vi "SLL Get Graph and File Sampling Rate.vi"(8 "error in (no error)":errorcluster) -> (0 "error out":errorcluster, 1 "File - Interval b/w Samples":i32, 2 "Graph - Interval b/w Samples":i32, 3 "AI Sampling Rate (Samples/Sec)":dbl)   [LabVIEW 2013]
doc: "Copyright © 2005, Soliton Technologies.\nAll rights reserved."
uses:
  DAQ Engine/Controls/SLL DE DAQ Parameters LV2Global Options.ctl
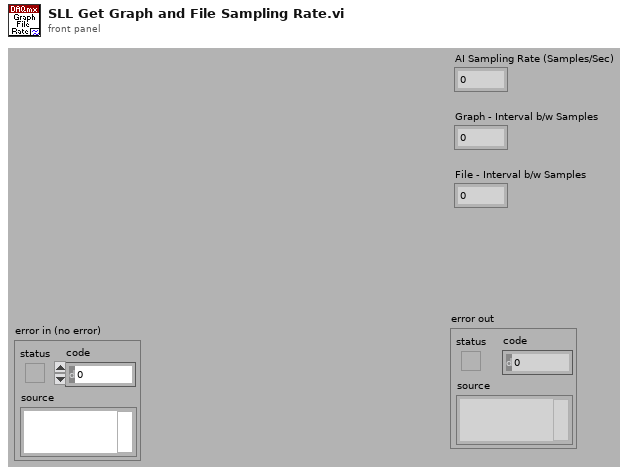
[diagram p1: front panel]
types:
  T1 = typedef "SLL DE DAQ Parameters LV2Global Options.ctl" = enum16{"Read", "Write"}
  T2 = typedef "SLL DE DAQ Engine Parameters.ctl" = cluster{"Enable Engines":cluster{"AI Enable":bool, "AO Enable":bool, "DI Enable":bool, "DO Enable":bool}, "DAQ Control Type":cluster{"Analog Input":enum16{"Finite", "Continuous", "Driver"}, "Analog Output":enum16{"Finite", "Continuous", "Driver"}, "Digital Input":enum16{"Finite", "Continuous", "Driver"}, "Digital Output":enum16{"Finite", "Continuous", "Driver"}}, "DAQ Parameters":cluster{"AI Sampling Rate (Samples/Sec)":dbl, "MvgAVG Window Size (# of Points)":i32, "Enable Filter":bool, "Enable MvgAVG":bool, "Circular Buffer Size (Sec)":dbl, "AO Sampling Rate (Samples/Sec)":dbl, "Graph Update Rate (Samples/Sec)":dbl, "File Logging Rate (Samples/Sec)":i32}, "AO Safe Values":cluster{"Analog Outputs Name":T3, "Analog Outputs Safe Value":dbl}[], "DO Safe Values":cluster{"Digital Outputs Name":T4, "Digital Outputs Safe Value":bool}[], "DO Interconnected Lines":cluster{"First DO Line":string, "Second DO Line":string}[], "AI Channels Unit":cluster{"Channel Name":T5, "Channel Type":T6}[], "Units Information":cluster{"Channel Type":T6, "Unit Text":string, "Maximum":dbl, "Minmum":dbl, "Increments":dbl}[]}
  T3 = typedef "SLL DE List of Analog Outputs.ctl" = enum16{"None"}
  T4 = typedef "SLL DE List of Digital Outputs.ctl" = enum16{"STATION1_START TEST", "STATION1_STOP TEST", "STATION1_LIGHT1", "STATION1_LIGHT2", "STATION1_LIGHT3", "STATION1_SELECT_TEST", "STATION2_START TEST", "STATION2_STOP TEST", "STATION2_LIGHT1", "STATION2_LIGHT2", "STATION2_LIGHT3", "STATION2_SELECT_TEST", "STATION3_START TEST", "STATION3_STOP TEST", "STATION3_LIGHT1", "STATION3_LIGHT2", "STATION3_LIGHT3", "STATION3_SELECT_TEST", "STATION4_START TEST", "STATION4_STOP TEST", "STATION4_LIGHT1", "STATION4_LIGHT2", "STATION4_LIGHT3", "STATION4_SELECT_TEST"}
  T5 = typedef "SLL DE List of Analog Inputs.ctl" = enum16{"None"}
  T6 = typedef "SLL DE List of AI Channel Type.ctl" = enum16{"Pressure", "Flow", "Temperature", "Time Scale", "Voltage", "Current", "Frequency", "Sound", "Speed", "Torque", "Distance", "Channel Type 1", "Channel Type 2", "Channel Type 3"}
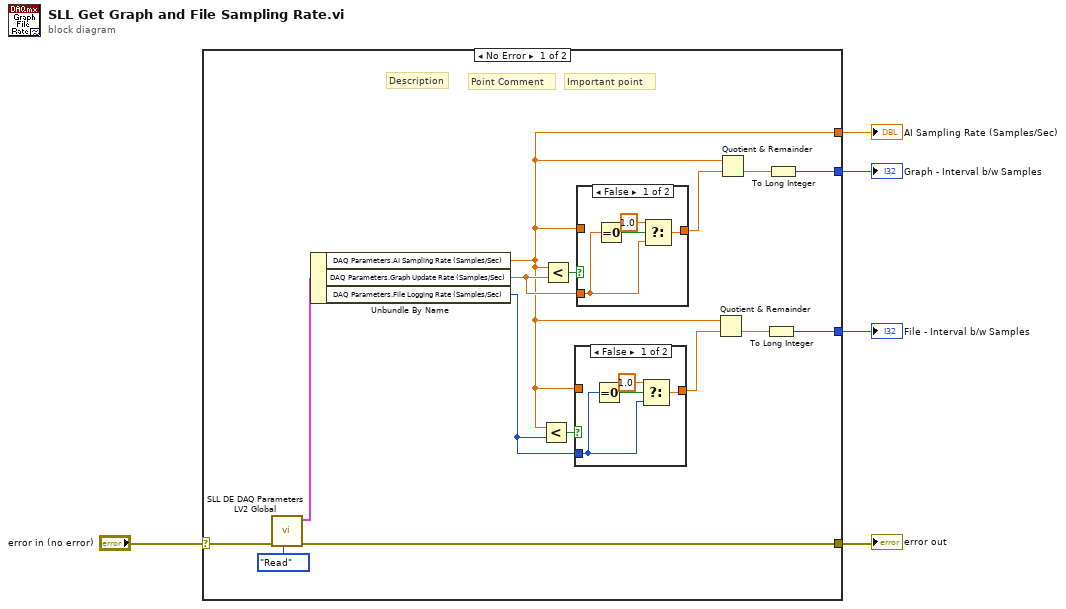
[diagram p0: block diagram]
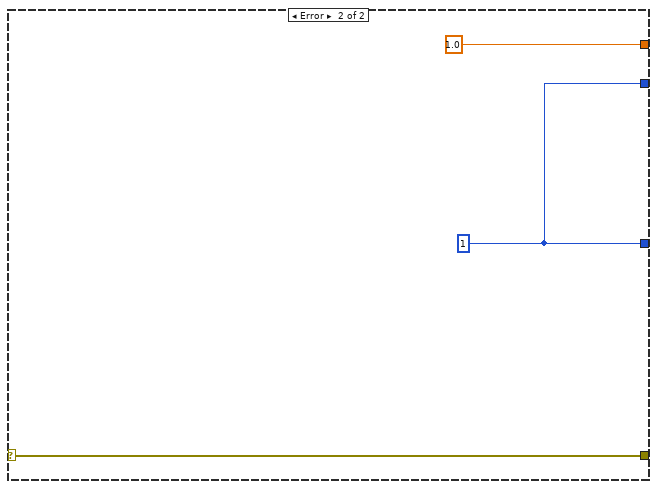
[diagram p4: hidden frame]
diagram:
  n1 = case shown="No Error" "error in (no error)" {
    selector: "error in (no error)" -> [w14 w33]
    tunnel: [w13 w33] -> w4
    tunnel: [w8 1.0 ("AI Sampling Rate (Samples/Sec)")] -> w3
    tunnel: [w7 w32] -> w2
    tunnel: [w6 w32] -> w1
    frame No Error {
      # "Point Comment"
      # "Important point"
      # "Description"
      n2 = call "SLL DE DAQ Parameters LV2 Global.vi"("Option"=SLL_DE_DAQ_Parameters_LV2Global_Options."Read", "Error in (no error)"=w14) -> ("Error out"=w13:errorcluster, "Global Info"=w17:T2)  [unwired: 8 in]
      n3 = Unbundle By Name(w17) -> ("DAQ Parameters.AI Sampling Rate (Samples/Sec)"=w8:dbl, "DAQ Parameters.Graph Update Rate (Samples/Sec)"=w19:dbl, "DAQ Parameters.File Logging Rate (Samples/Sec)"=w9:i32)
      n4 = Less?(x=w8, y=w9) -> (x < y?=w12:bool)
      n5 = Less?(x=w8, y=w19) -> (x < y?=w15:bool)
      n6 = case shown="False" w12 {
        tunnel: [w24 w25] -> w10
        tunnel: w8 -> [_ w25]
        tunnel: w9 -> [w21 _]
        frame False {
          n7 = Equal To 0?(x=w21) -> (x = 0?=w23:bool)
          n8 = Select(t=1.0, s=w23, f=w21) -> (s? t:f=w24:dbl)
        }
        frame True {
        }
      }
      n9 = case shown="False" w15 {
        tunnel: [w29 w30] -> w20
        tunnel: w8 -> [_ w30]
        tunnel: w19 -> [w26 _]
        frame False {
          n10 = Equal To 0?(x=w26) -> (x = 0?=w28:bool)
          n11 = Select(t=1.0, s=w28, f=w26) -> (s? t:f=w29:dbl)
        }
        frame True {
        }
      }
      n12 = Quotient & Remainder(x=w8, y=w10) -> (floor(x/y)=w11:dbl)  [unwired: 1 out]
      n13 = Quotient & Remainder(x=w8, y=w20) -> (floor(x/y)=w18:dbl)  [unwired: 1 out]
      n14 = To Long Integer(number=w11) -> (32bit integer=w6:i32)
      n15 = To Long Integer(number=w18) -> (32bit integer=w7:i32)
    }
    frame Error {
      w32 = 1
    }
  }
  "error out" <- w4
  "AI Sampling Rate (Samples/Sec)" <- w3
  "Graph - Interval b/w Samples" <- w2
  "File - Interval b/w Samples" <- w1
